vi "Create User Event - Stop.vi"(8 "error in":errorcluster) -> (0 "error out":errorcluster, 2 "User Event - Stop":refnum<user-event>, 3 "Stop Event Registration Refnum":refnum<event-registration>)   [LabVIEW 2022 SP3, in "User Event - Stop.lvlib"]
doc: "Create a boolean user event that will be used to stop the event loop from the message handling loop."
uses:
  User Event - Stop.lvlib
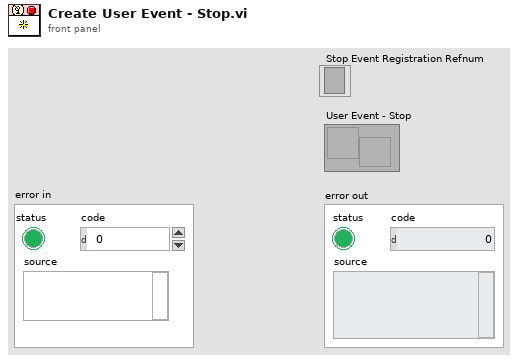
[diagram p1: front panel]
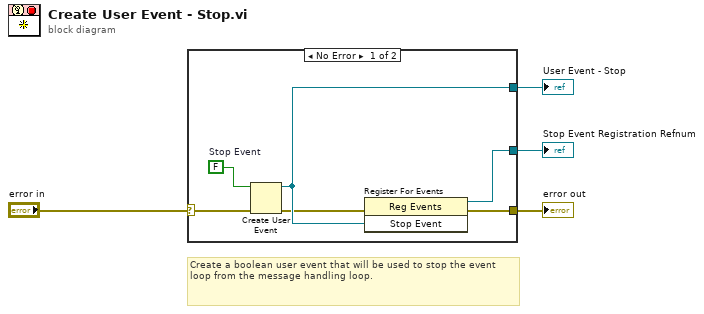
[diagram p0: block diagram]
diagram:
  # "Create a boolean user event that will be used to stop the event loop from the message handling loop."
  n1 = case shown="No Error" "error in" {
    selector: "error in" -> [w5 w11]
    tunnel: [w10 _] -> w4
    tunnel: [w9 _] -> w3
    tunnel: [w6 w11] -> w1
    frame No Error {
      w8 = FALSE  # Stop Event
      n2 = Create User Event(user event datatype=w8, error in=w5) -> (user event=w10:refnum<user-event>, error out=w7:errorcluster)
      n3 = register-events(error in=w7, w10) -> (reference out=w9:refnum<event-registration>, error out=w6:errorcluster)  [unwired: 1 in]
    }
    frame Error {
    }
  }
  "User Event - Stop" <- w4
  "Stop Event Registration Refnum" <- w3
  "error out" <- w1
